vi "Hash.vi"(8 "error in (no error)":errorcluster, 10 "Message":string, 11 "Hash in":refnum<class "Hash.lvclass">) -> (0 "error out":errorcluster, 2 "Hash":string, 3 "Hash out":refnum<class "Hash.lvclass">)   [LabVIEW 2015, in "Crypto.lvlib" / "Hash.lvclass"]
uses:
  Hash.lvclass
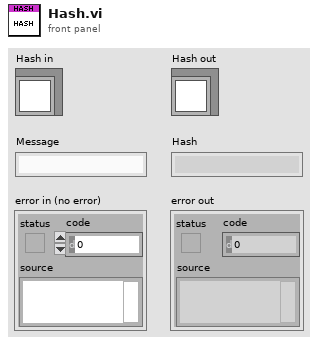
[diagram p1: front panel]
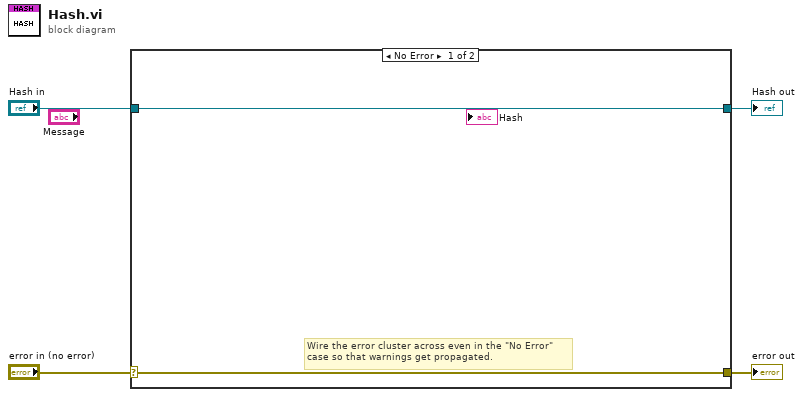
[diagram p0: block diagram]
diagram:
  n1 = case shown="No Error" "error in (no error)" {
    selector: "error in (no error)" -> [w5 w8]
    tunnel: [w5 w8] -> w3
    tunnel: [w6 w7] -> w1
    tunnel: "Hash in" -> [w6 w7]
    frame No Error {
      # "Wire the error cluster across even in the \"No Error\"\ncase so that warnings get propagated."
    }
    frame Error {
    }
  }
  "error out" <- w3
  "Hash out" <- w1
